vi "BetterNumeric.vi"(1 "stop":bool, 2 "BetterNumeric in":T1 {"Value" step=1e-50}) -> (0 "BetterNumeric out":T1 {"Value" step=1e-50})   [LabVIEW 2013]
uses:
  Controls/BetterNumeric.ctl
panel:
  in  "Inc/Dec by 0.1 Barrier":u8=2 min=1 max=10 step=1
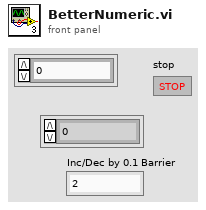
[diagram p1: front panel]
types:
  T1 = typedef "BetterNumeric.ctl" = cluster{"Value":dbl, "Down":bool, "Up":bool}
  T2 = typedef "eventvkey.ctl" = enum16{"ASCII", "Enter", "Return", "Shift", "Ctrl", "Alt", "Cmd", "Opt", "Caps", "NumLock", "Clear", "Break", "Up", "Down", "Left", "Right", "Insert", "Delete", "Home", "End", "PageUp", "PageDown", "Escape", "Help", "Pause", "ScrollLock", "F1", "F2", "F3", "F4", "F5", "F6", "F7", "F8", "F9", "F10", "F11", "F12", "F13", "F14", "F15", "F16", "F17", "F18", "F19", "F20", "F21", "F22", "F23", "F24", "Play", "VolumeUp", "VolumeDown", "Mute", "Two Byte Char"}
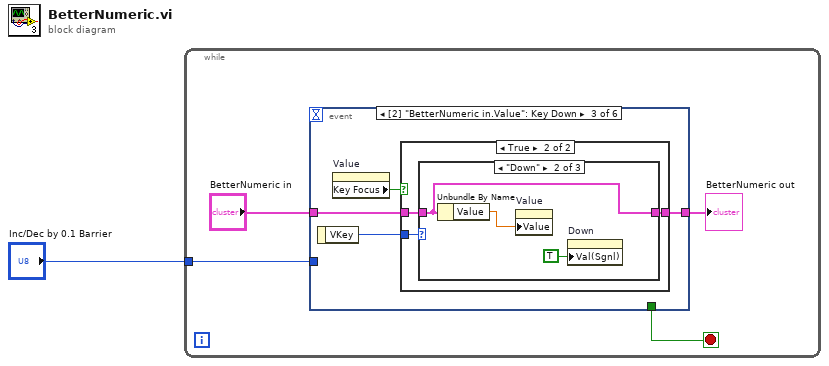
[diagram p0: block diagram]
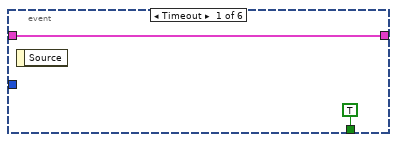
[diagram p2: hidden frame]
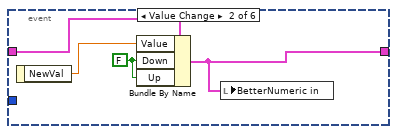
[diagram p3: hidden frame]
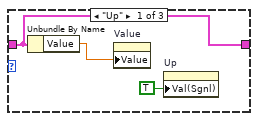
[diagram p5: hidden frame]
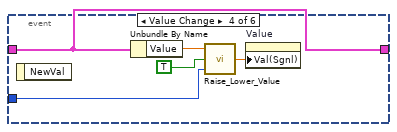
[diagram p7: hidden frame]
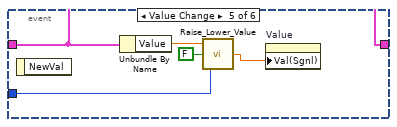
[diagram p8: hidden frame]
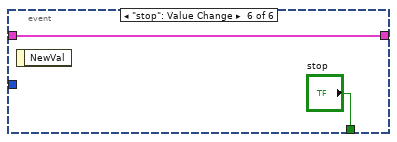
[diagram p9: hidden frame]
diagram:
  n1 = while {
    tunnel: "Inc/Dec by 0.1 Barrier" -> [w2]
    stop <- w5 stop-if-true
    n2 = event shown="[2] \"BetterNumeric in.Value\": Key Down" {
      selector: _ -> [_ _ _ _ _ _]
      dyn-events: _ -> [_ _ _ _ _ _]
      timeout: _ -> [_ _ _ _ _ _]
      tunnel: "BetterNumeric in" -> [w7 w11 w13 w31 w36 w37]
      tunnel: [w7 w8 w12 w31 w36 w37] -> w3
      tunnel: [TRUE ("stop") _ _ _ _ "stop"] -> w5
      tunnel: w2 -> [_ _ _ w28 w32 _]
      event Timeout {
        n3 = event-data() -> ()  [unwired: 1 in, 1 out]
      }
      event Value Change {
        w9 = FALSE ("Down")
        n4 = event-data() -> ("NewVal"=w10:dbl)  [unwired: 1 in]
        n5 = Bundle By Name(cluster=w11, "Value"=w10, "Down"=w9, "Up"=w9) -> (w8:T1)
        n6 = local write "BetterNumeric in"(w8) -> ()
      }
      event Key Down {
        n7 = event-data() -> ("VKey"=w15:T2)  [unwired: 1 in]
        n8 = property on="Value" class="DigNum (strict)"() -> ("Key Focus"=w14:bool)  [unwired: 2 in, 2 out]
        n9 = case shown="True" w14 {
          tunnel: w15 -> [_ w19]
          tunnel: w13 -> [w16 w18]
          tunnel: [w16 w17] -> w12
          frame False {
          }
          frame True {
            n10 = case shown="\"Down\"" w19 {
              tunnel: w18 -> [w22 w25 w26]
              tunnel: [w22 w25 w26] -> w17
              frame "Up" {
                n11 = Unbundle By Name(w22) -> ("Value"=w20:dbl)
                n12 = property on="Value" class="DigNum (strict)"("Value"=w20) -> ()  [unwired: 2 in, 2 out]
                n13 = property on="Up" class="Bool (strict)"("Val(Sgnl)"=TRUE ("Value (Signaling)")) -> ()  [unwired: 2 in, 2 out]
              }
              frame "Down" {
                n14 = Unbundle By Name(w25) -> ("Value"=w23:dbl)
                n15 = property on="Value" class="DigNum (strict)"("Value"=w23) -> ()  [unwired: 2 in, 2 out]
                n16 = property on="Down" class="Bool (strict)"("Val(Sgnl)"=TRUE ("Value (Signaling)")) -> ()  [unwired: 2 in, 2 out]
              }
              frame "ASCII", Default {
              }
            }
          }
        }
      }
      event Value Change {
        n17 = event-data() -> ()  [unwired: 1 in, 1 out]
        n18 = Unbundle By Name(w31) -> ("Value"=w30:dbl)
        n19 = call "Raise_Lower_Value.vi"("Inc/Dec by 0.1 Barrier"=w28, "Raise Value?"=TRUE, "Value in"=w30) -> ("Value out"=w27:dbl)
        n20 = property on="Value" class="DigNum (strict)"("Val(Sgnl)"=w27) -> ()  [unwired: 2 in, 2 out]
      }
      event Value Change {
        n21 = event-data() -> ()  [unwired: 1 in, 1 out]
        n22 = Unbundle By Name(w36) -> ("Value"=w35:dbl)
        n23 = call "Raise_Lower_Value.vi"("Inc/Dec by 0.1 Barrier"=w32, "Raise Value?"=FALSE, "Value in"=w35) -> ("Value out"=w33:dbl)
        n24 = property on="Value" class="DigNum (strict)"("Val(Sgnl)"=w33) -> ()  [unwired: 2 in, 2 out]
      }
      event "stop": Value Change {
        n25 = event-data() -> ()  [unwired: 1 in, 1 out]
      }
    }
    "BetterNumeric out" <- w3
  }
